vi "test - filter JKISM String Queue.vi"(8 "error in (no error)":errorcluster, 11 "TestCase in":refnum<class "testcase-Basic-Function.lvclass">) -> (0 "error out":errorcluster, 3 "TestCase out":refnum<class "testcase-Basic-Function.lvclass">)   [LabVIEW 2017, in "testcase-Basic-Function.lvclass"]
uses:
  testcase-Basic-Function.lvclass
  src/user.lib/_NEVSTOP/Communicable State Machine(CSM)/_Polymophic/CSM - Filter Broadcasts.vi
  src/user.lib/_NEVSTOP/Communicable State Machine(CSM)/_Polymophic/CSM - Filter Interrupt Broadcasts.vi
  src/user.lib/_NEVSTOP/Communicable State Machine(CSM)/_Polymophic/CSM - Filter Status Broadcasts.vi
  src/user.lib/_NEVSTOP/Communicable State Machine(CSM)/AdvanceAPI/CSM - Filter Messages to Non-Existing Modules.vi
  src/user.lib/_NEVSTOP/Communicable State Machine(CSM)/_Polymophic/CSM - Filter Sync Messages.vi
  src/user.lib/_NEVSTOP/Communicable State Machine(CSM)/_Polymophic/CSM - Filter Async without Reply Messages.vi
  src/user.lib/_NEVSTOP/Communicable State Machine(CSM)/_Polymophic/CSM - Filter Async Messages.vi
  src/user.lib/_NEVSTOP/Communicable State Machine(CSM)/_Polymophic/CSM - Filter Messges.vi
  src/user.lib/_NEVSTOP/Communicable State Machine(CSM)/_Polymophic/CSM - Filter Local States.vi
  src/user.lib/_NEVSTOP/Communicable State Machine(CSM)/_Polymophic/CSM - Filter Duplicated Lines.vi
  <vilib>/addons/_JKI Toolkits/VI Tester/TestCase.llb/TestCase.lvclass
  src/user.lib/_NEVSTOP/Communicable State Machine(CSM)/Communicable State Machine.lvlib
  C:/Program Files (x86)/National Instruments/LabVIEW 2017/vi.lib/addons/_JKI Toolkits/VI Tester/TestCase.llb/TestCase.lvclass
panel:
  out "MONITOR":errorcluster[](array[cluster])
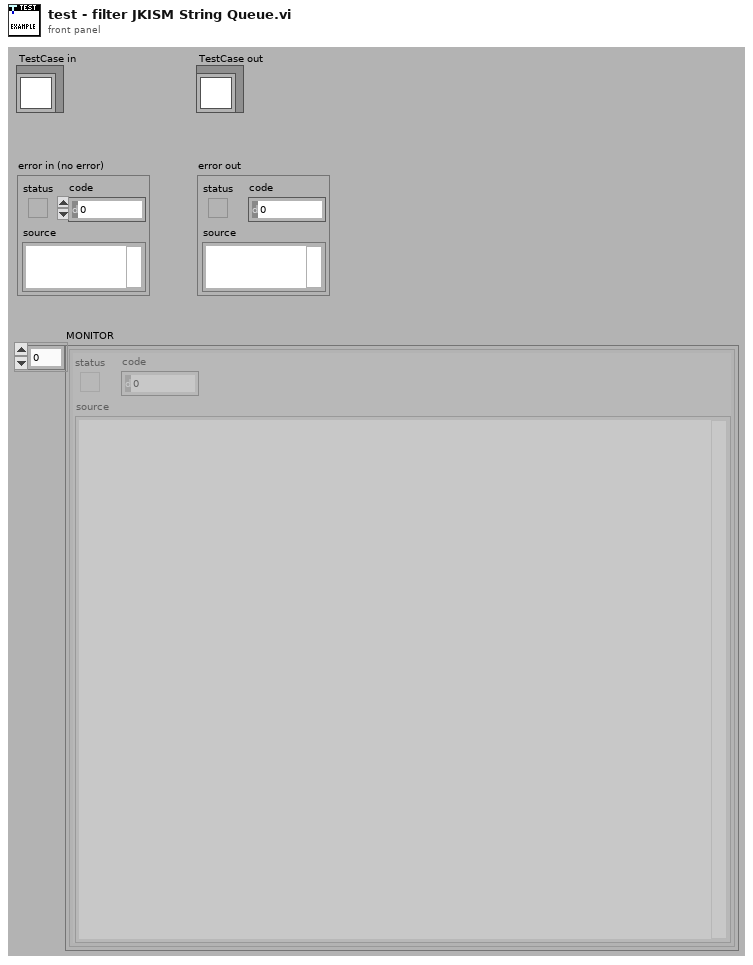
[diagram p1: front panel]
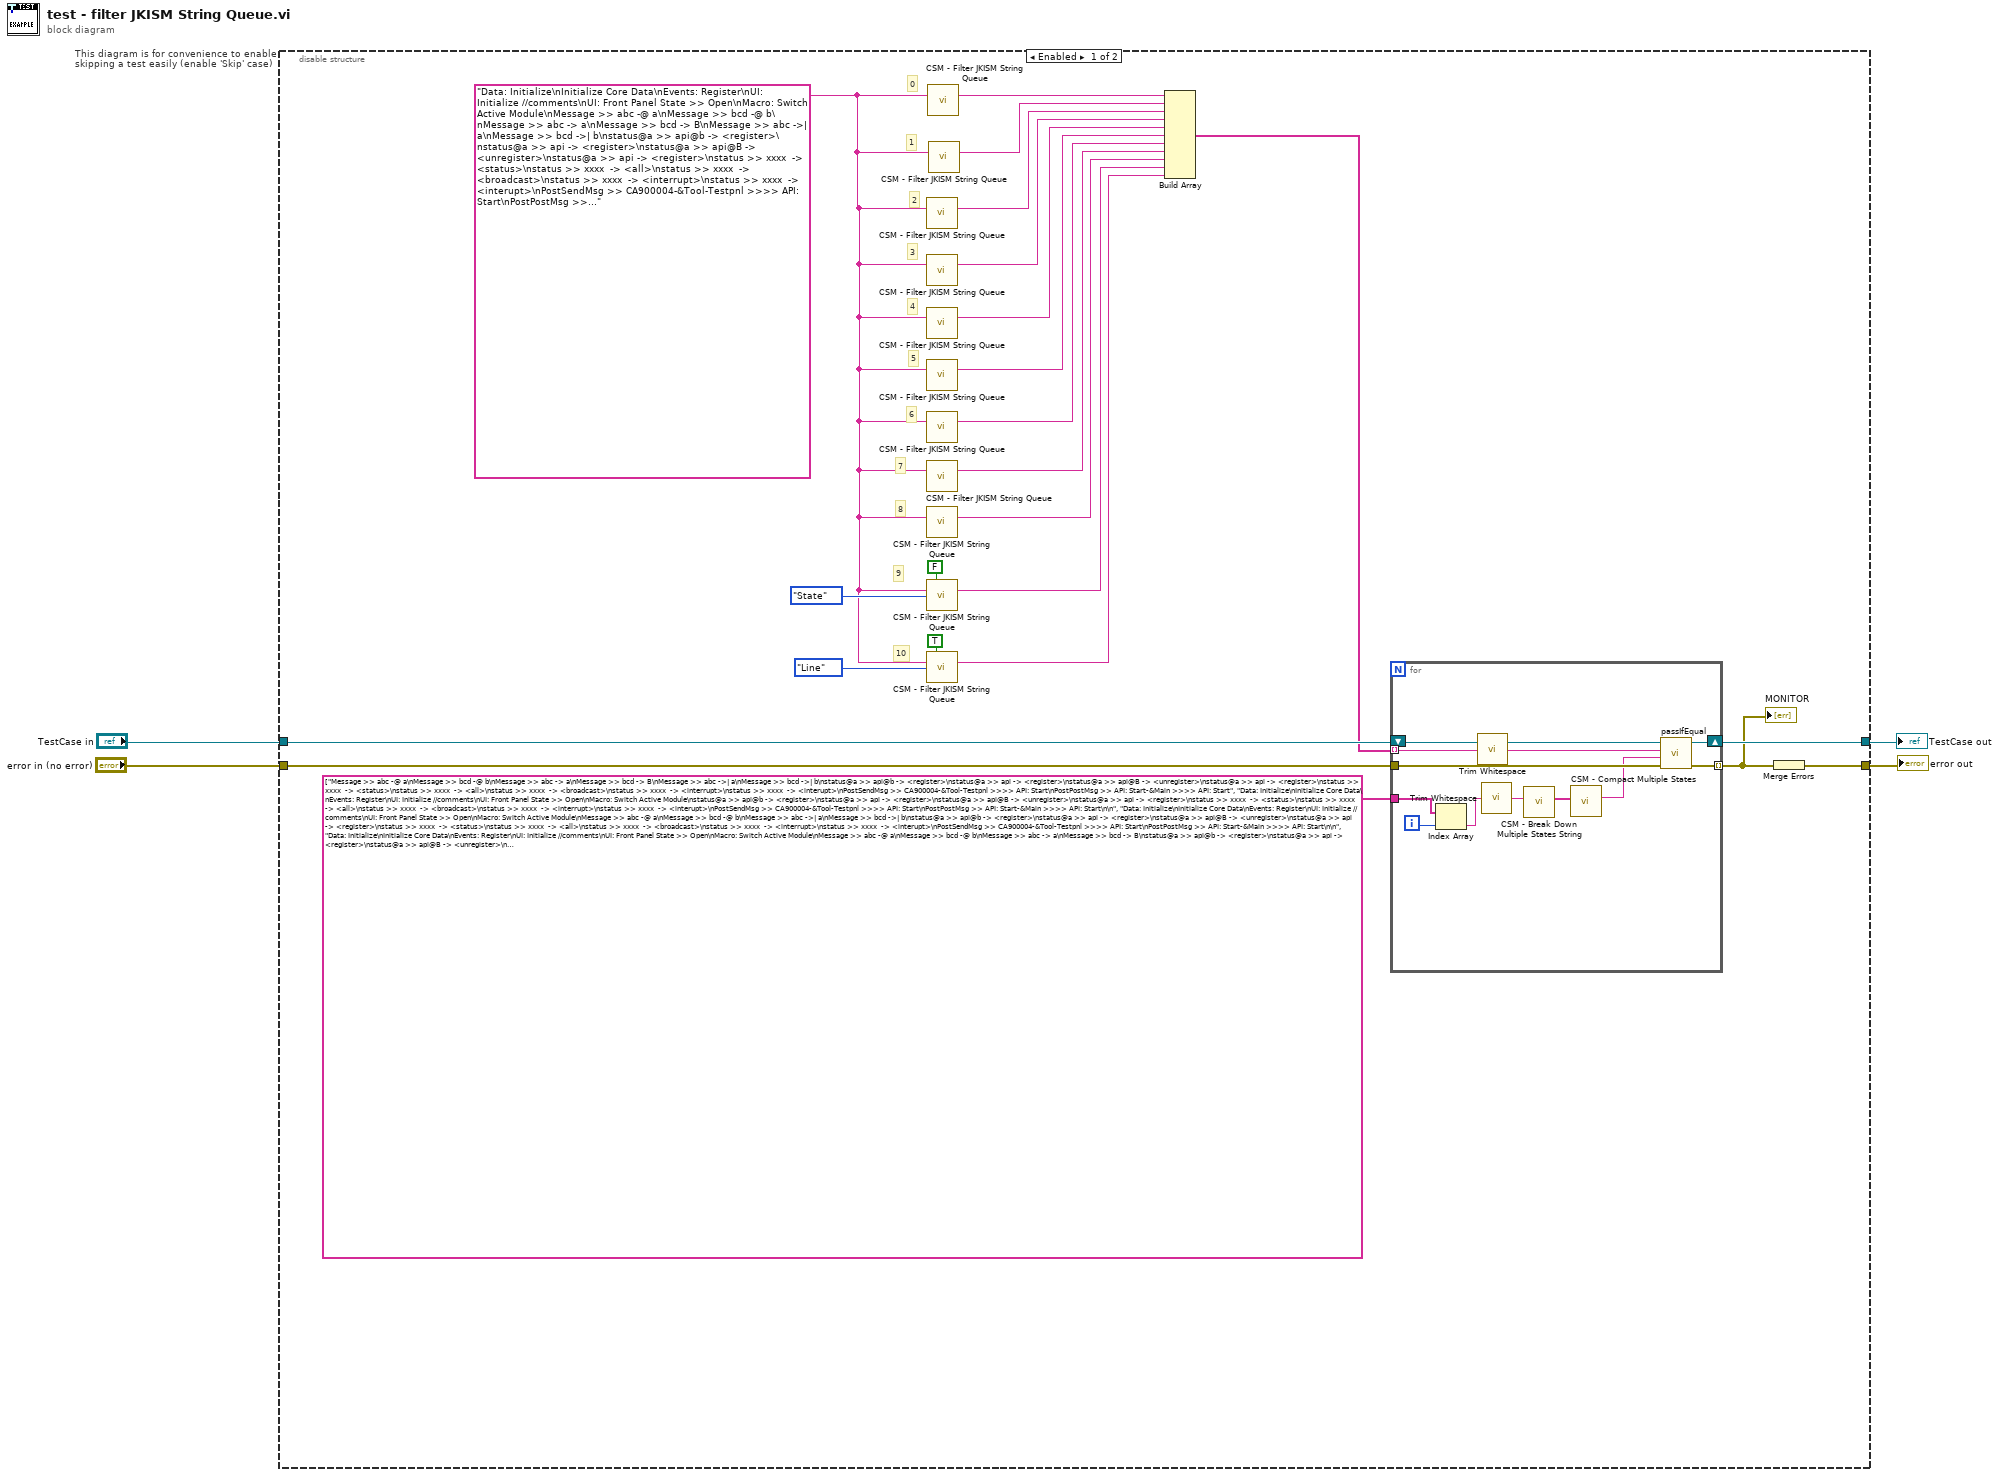
[diagram p0: block diagram]
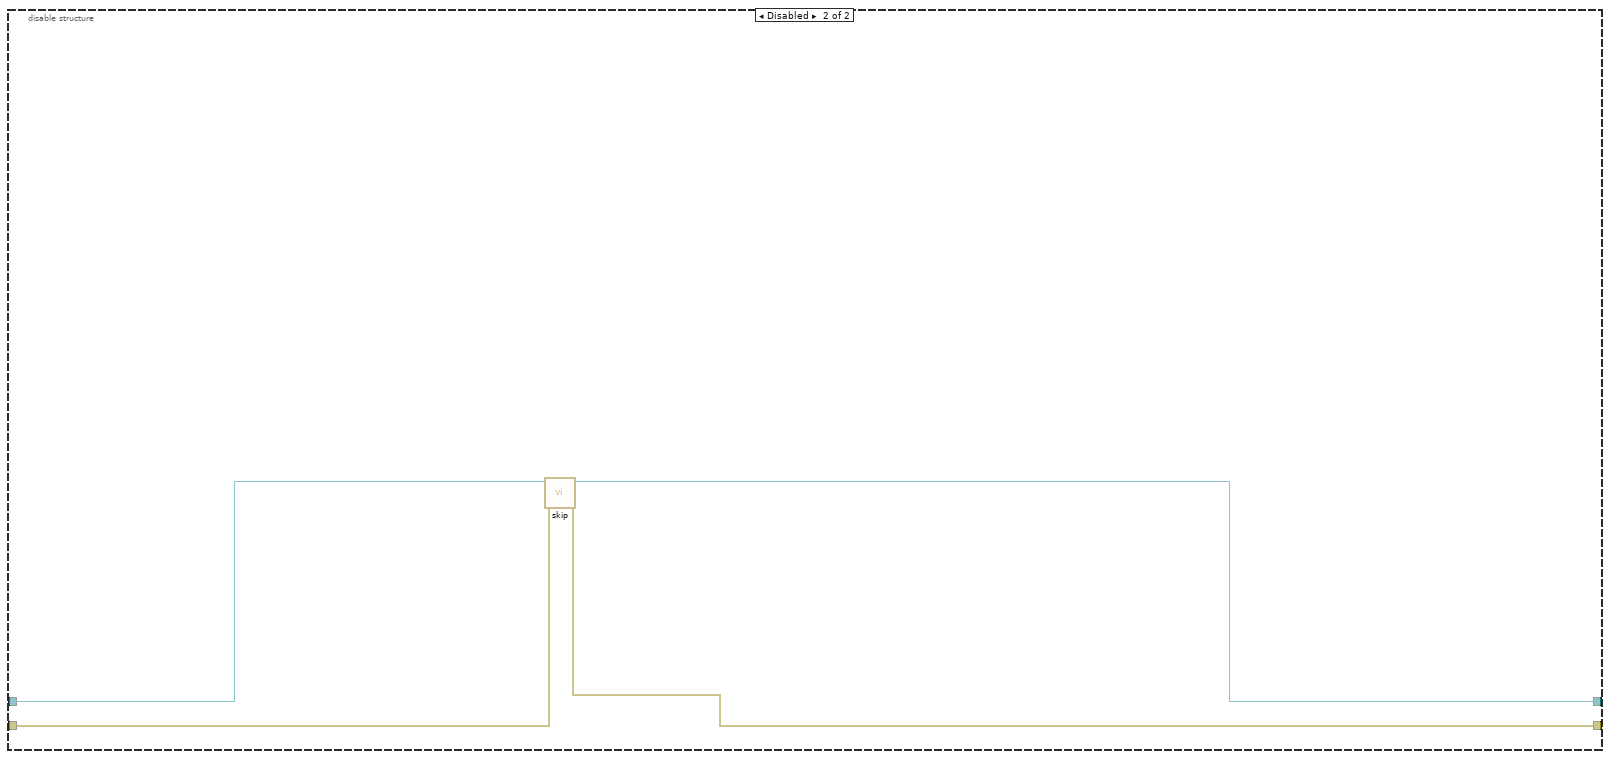
[diagram p2: hidden frame]
diagram:
  n1 = disable-structure "This diagram is for convenience to enable skipping a test easily (enable 'Skip' case)" shown="Enabled" {
    disable-tunnel: "TestCase in" -> [w27 w43]
    disable-tunnel: [w23 w41] -> w1
    disable-tunnel: [w17 w42] -> w3
    disable-tunnel: "error in (no error)" -> [w26 w40]
    frame Enabled {
      w8 = "Data: Initialize\nInitialize Core Data\nEvents: Register\nUI: Initialize //comments\nUI: Front Panel State >> Open\nMacro: Switch Active Module\nMessage >> abc -@ a\nMessage >> bcd -@ b\nMessage >> abc -> a\nMessage >> bcd -> B\nMessage >> abc ->| a\nMessage >> bcd ->| b\nstatus@a >> api@b -> <register>\nstatus@a >> api -> <register>\nstatus@a >> api@B -> <unregister>\nstatus@a >> api -> <register>\nstatus >> xxxx  -> <status>\nstatus >> xxxx  -> <all>\nstatus >> xxxx  -> <broadcast>\nstatus >> xxxx  -> <interrupt>\nstatus >> xxxx  -> <interupt>\nPostSendMsg >> CA900004-&Tool-Testpnl >>>> API: Start\nPostPostMsg >> API: Start-&Main >>>> API: Start\n" ("States")
      # "10"
      # "9"
      # "8"
      # "7"
      # "6"
      # "5"
      # "4"
      # "3"
      # "2"
      # "1"
      # "0"
      n2 = call-poly "CSM - Filter JKISM String Queue.vi"("State(s) in (\"\")"=w8) -> ("States Out"=w20:string)  [unwired: 14 in]
      n3 = call-poly "CSM - Filter JKISM String Queue.vi"("State(s) in (\"\")"=w8) -> ("States Out"=w19:string)  [unwired: 14 in]
      n4 = call-poly "CSM - Filter JKISM String Queue.vi"("State(s) in (\"\")"=w8) -> ("States Out"=w18:string)  [unwired: 14 in]
      n5 = call-poly "CSM - Filter JKISM String Queue.vi"("State(s) in (\"\")"=w8) -> ("States Out"=w16:string)  [unwired: 14 in]
      n6 = call-poly "CSM - Filter JKISM String Queue.vi"("State(s) in (\"\")"=w8) -> ("States Out"=w14:string)  [unwired: 14 in]
      n7 = call-poly "CSM - Filter JKISM String Queue.vi"("State(s) in (\"\")"=w8) -> ("States Out"=w13:string)  [unwired: 14 in]
      n8 = call-poly "CSM - Filter JKISM String Queue.vi"("State(s) in (\"\")"=w8) -> ("States Out"=w12:string)  [unwired: 14 in]
      n9 = call-poly "CSM - Filter JKISM String Queue.vi"("Keep First Matched?(T)"=FALSE, "State(s) in (\"\")"=w8, "Option"=enum16{"State", "No Comments", "Line"}."State") -> ("States Out"=w11:string)  [unwired: 12 in]
      n10 = call-poly "CSM - Filter JKISM String Queue.vi"("Keep First Matched?(T)"=TRUE, "State(s) in (\"\")"=w8, "Option"=enum16{"State", "No Comments", "Line"}."Line") -> ("States Out"=w7:string)  [unwired: 12 in]
      n11 = call-poly "CSM - Filter JKISM String Queue.vi"("State(s) in (\"\")"=w8) -> ("States Out"=w24:string)  [unwired: 14 in]
      n12 = call-poly "CSM - Filter JKISM String Queue.vi"("State(s) in (\"\")"=w8) -> ("States Out"=w21:string)  [unwired: 14 in]
      n13 = Build Array(w24, w21, w20, w19, w18, w16, w14, w13, w12, w11, w7) -> (w22:string[])
      n14 = for {
        tunnel: string[] ["Message >> abc -@ a\nMessage >> bcd -@ b\nMessage >> abc -> a\nMessage >> bcd -> B\nMessage >> abc ->| a\nMessage >> bcd ->| b\nstatus@a >> api@b -> <register>\nstatus@a >> api -> <register>\nstatus@a >> api@B -> <unregister>\nstatus@a >> api -> <register>\nstatus >> xxxx  -> <status>\nstatus >> xxxx  -> <all>\nstatus >> xxxx  -> <broadcast>\nstatus >> xxxx  -> <interrupt>\nstatus >> xxxx  -> <interupt>\nPostSendMsg >> CA900004-&Tool-Testpnl >>>> API: Start\nPostPostMsg >> API: Start-&Main >>>> API: Start", "Data: Initialize\nInitialize Core Data\nEvents: Register\nUI: Initialize //comments\nUI: Front Panel State >> Open\nMacro: Switch Active Module\nstatus@a >> api@b -> <register>\nstatus@a >> api -> <register>\nstatus@a >> api@B -> <unregister>\nstatus@a >> api -> <register>\nstatus >> xxxx  -> <status>\nstatus >> xxxx  -> <all>\nstatus >> xxxx  -> <broadcast>\nstatus >> xxxx  -> <interrupt>\nstatus >> xxxx  -> <interupt>\nPostSendMsg >> CA900004-&Tool-Testpnl >>>> API: Start\nPostPostMsg >> API: Start-&Main >>>> API: Start\n\n", "Data: Initialize\nInitialize Core Data\nEvents: Register\nUI: Initialize //comments\nUI: Front Panel State >> Open\nMacro: Switch Active Module\nMessage >> abc -@ a\nMessage >> bcd -@ b\nMessage >> abc ->| a\nMessage >> bcd ->| b\nstatus@a >> api@b -> <register>\nstatus@a >> api -> <register>\nstatus@a >> api@B -> <unregister>\nstatus@a >> api -> <register>\nstatus >> xxxx  -> <status>\nstatus >> xxxx  -> <all>\nstatus >> xxxx  -> <broadcast>\nstatus >> xxxx  -> <interrupt>\nstatus >> xxxx  -> <interupt>\nPostSendMsg >> CA900004-&Tool-Testpnl >>>> API: Start\nPostPostMsg >> API: Start-&Main >>>> API: Start\n\n", "Data: Initialize\nInitialize Core Data\nEvents: Register\nUI: Initialize //comments\nUI: Front Panel State >> Open\nMacro: Switch Active Module\nMessage >> abc -@ a\nMessage >> bcd -@ b\nMessage >> abc -> a\nMessage >> bcd -> B\nstatus@a >> api@b -> <register>\nstatus@a >> api -> <register>\nstatus@a >> api@B -> <unregister>\nstatus@a >> api -> <register>\nstatus >> xxxx  -> <status>\nstatus >> xxxx  -> <all>\nstatus >> xxxx  -> <broadcast>\nstatus >> xxxx  -> <interrupt>\nstatus >> xxxx  -> <interupt>\nPostSendMsg >> CA900004-&Tool-Testpnl >>>> API: Start\nPostPostMsg >> API: Start-&Main >>>> API: Start", "Data: Initialize\nInitialize Core Data\nEvents: Register\nUI: Initialize //comments\nUI: Front Panel State >> Open\nMacro: Switch Active Module\nMessage >> abc -> a\nMessage >> bcd -> B\nMessage >> abc ->| a\nMessage >> bcd ->| b\nstatus@a >> api@b -> <register>\nstatus@a >> api -> <register>\nstatus@a >> api@B -> <unregister>\nstatus@a >> api -> <register>\nstatus >> xxxx  -> <status>\nstatus >> xxxx  -> <all>\nstatus >> xxxx  -> <broadcast>\nstatus >> xxxx  -> <interrupt>\nstatus >> xxxx  -> <interupt>\nPostSendMsg >> CA900004-&Tool-Testpnl >>>> API: Start\nPostPostMsg >> API: Start-&Main >>>> API: Start", "Data: Initialize\nInitialize Core Data\nEvents: Register\nUI: Initialize //comments\nUI: Front Panel State >> Open\nMacro: Switch Active Module\nstatus@a >> api@b -> <register>\nstatus@a >> api -> <register>\nstatus@a >> api@B -> <unregister>\nstatus@a >> api -> <register>\nstatus >> xxxx  -> <status>\nstatus >> xxxx  -> <all>\nstatus >> xxxx  -> <broadcast>\nstatus >> xxxx  -> <interrupt>\nstatus >> xxxx  -> <interupt>\nPostSendMsg >> CA900004-&Tool-Testpnl >>>> API: Start\nPostPostMsg >> API: Start-&Main >>>> API: Start", "Data: Initialize\nInitialize Core Data\nEvents: Register\nUI: Initialize //comments\nUI: Front Panel State >> Open\nMacro: Switch Active Module\nMessage >> abc -@ a\nMessage >> bcd -@ b\nMessage >> abc -> a\nMessage >> bcd -> B\nMessage >> abc ->| a\nMessage >> bcd ->| b\nstatus@a >> api@b -> <register>\nstatus@a >> api -> <register>\nstatus@a >> api@B -> <unregister>\nstatus@a >> api -> <register>\nstatus >> xxxx  -> <interrupt>\nstatus >> xxxx  -> <interupt>\nPostSendMsg >> CA900004-&Tool-Testpnl >>>> API: Start\nPostPostMsg >> API: Start-&Main >>>> API: Start", "Data: Initialize\nInitialize Core Data\nEvents: Register\nUI: Initialize //comments\nUI: Front Panel State >> Open\nMacro: Switch Active Module\nMessage >> abc -@ a\nMessage >> bcd -@ b\nMessage >> abc -> a\nMessage >> bcd -> B\nMessage >> abc ->| a\nMessage >> bcd ->| b\nstatus@a >> api@b -> <register>\nstatus@a >> api -> <register>\nstatus@a >> api@B -> <unregister>\nstatus@a >> api -> <register>\nstatus >> xxxx  -> <status>\nstatus >> xxxx  -> <all>\nstatus >> xxxx  -> <broadcast>\nPostSendMsg >> CA900004-&Tool-Testpnl >>>> API: Start\nPostPostMsg >> API: Start-&Main >>>> API: Start", "Data: Initialize\nInitialize Core Data\nEvents: Register\nUI: Initialize //comments\nUI: Front Panel State >> Open\nMacro: Switch Active Module\nMessage >> abc -@ a\nMessage >> bcd -@ b\nMessage >> abc -> a\nMessage >> bcd -> B\nMessage >> abc ->| a\nMessage >> bcd ->| b\nstatus@a >> api@b -> <register>\nstatus@a >> api -> <register>\nstatus@a >> api@B -> <unregister>\nstatus@a >> api -> <register>\nPostSendMsg >> CA900004-&Tool-Testpnl >>>> API: Start\nPostPostMsg >> API: Start-&Main >>>> API: Start\n\n", "Data: Initialize\nInitialize Core Data\nEvents: Register\nUI: Initialize //comments\nUI: Front Panel State >> Open\nMacro: Switch Active Module\nMessage >> bcd ->| b\nstatus@a >> api -> <register>\nstatus >> xxxx  -> <interupt>\nPostSendMsg >> CA900004-&Tool-Testpnl >>>> API: Start\nPostPostMsg >> API: Start-&Main >>>> API: Start", "Data: Initialize\nInitialize Core Data\nEvents: Register\nUI: Initialize //comments\nUI: Front Panel State >> Open\nMacro: Switch Active Module\nMessage >> abc -@ a\nMessage >> bcd -@ b\nMessage >> abc -> a\nMessage >> bcd -> B\nMessage >> abc ->| a\nMessage >> bcd ->| b\nstatus@a >> api@b -> <register>\nstatus@a >> api -> <register>\nstatus@a >> api@B -> <unregister>\nstatus >> xxxx  -> <status>\nstatus >> xxxx  -> <all>\nstatus >> xxxx  -> <broadcast>\nstatus >> xxxx  -> <interrupt>\nstatus >> xxxx  -> <interupt>\nPostSendMsg >> CA900004-&Tool-Testpnl >>>> API: Start\nPostPostMsg >> API: Start-&Main >>>> API: Start"] ("States") -> [w29]
        tunnel: w22 -> [w37] mode=indexing
        shift-right: [w31] -> w23
        shift-left: w27 -> [w39]
        tunnel: w26 -> [w38]
        tunnel: [w32] -> w15 mode=indexing
        i -> [w30]
        n15 = Index Array(array=w29, index=w30) -> (element=w28:string)
        n16 = call <vilib>:"Trim Whitespace.vi"("string"=w37) -> ("trimmed string"=w36:string)  [unwired: 1 in]
        n17 = call <vilib>:"Trim Whitespace.vi"("string"=w28) -> ("trimmed string"=w34:string)  [unwired: 1 in]
        n18 = call "CSM - Break Down Multiple States String.vi"("States"=w34) -> ("Multiple States"=w35:string[])  [unwired: 10 in]
        n19 = call "CSM - Compact Multiple States.vi"("Multiple States"=w35) -> ("States"=w33:string)  [unwired: 9 in]
        n20 = call-dynamic "passIfEqual.vi"("error in (no error)"=w38, "y"=w33, "x"=w36, "TestCase in"=w39) -> ("error out"=w32:errorcluster, "TestCase out"=w31:refnum<class "testcase-Basic-Function.lvclass">)  [unwired: 6 in]
      }
      "MONITOR" <- w15
      n21 = Merge Errors(w15) -> (w17:errorcluster)
    }
    frame Disabled {
      # "skip test result while test is under development"
      n22 = call <vilib>:"skip.vi"("error in (no error)"=w40, "TestCase in"=w43) -> ("error out"=w42:errorcluster, "TestCase out"=w41:refnum<class "testcase-Basic-Function.lvclass">)  [unwired: 8 in]
    }
  }
  "error out" <- w3
  "TestCase out" <- w1
